vi "MB Write Coil.vi"(8 "error in (no error)":errorcluster, 9 "Key":string="Servodriver_On", 10 "Write Value":bool, 11 "Devices":T1) -> (0 "error out":errorcluster, 3 "Devices Out":T1)   [LabVIEW 2021]
uses:
  Modbus Cluster.ctl
  <vilib>/NI/Modbus Library/API/Master/Modbus Master.lvclass
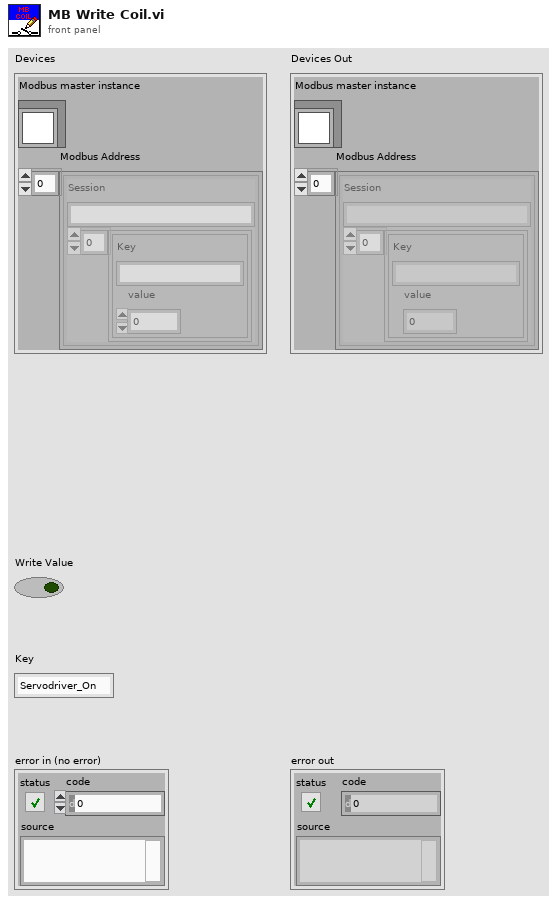
[diagram p1: front panel]
types:
  T1 = typedef "Modbus Cluster.ctl" = cluster{"Modbus master instance":refnum<class "Modbus Master.lvclass">, "Modbus Address":cluster{"Session":string, cluster{"Key":string, "value":u32}[]}[]}
  T2 = cluster{"Session":string, cluster{"Key":string, "value":u32}[]}[]
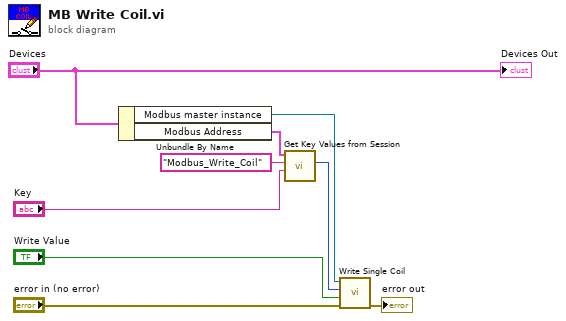
[diagram p0: block diagram]
diagram:
  n1 = Unbundle By Name("Devices") -> ("Modbus master instance"=w9:refnum<class "Modbus Master.lvclass">, "Modbus Address"=w2:T2)
  n2 = call "Get Key Values from Session.vi"("Key"="Key", "Session"="Modbus_Write_Coil", "Ini File"=w2) -> ("Search Key Value"=w3:u32)  [unwired: 6 in, 2 out]
  n3 = call-dynamic "Write Single Coil.vi"("error in"="error in (no error)", "coil to write"="Write Value", "address"=w3, "Modbus master in"=w9) -> ("error out"=→"error out":errorcluster)  [unwired: 6 in, 1 out]
  "Devices Out" <- "Devices"
